vi "XML - Get extra pages XML string.vi"(8 "error in (no error)":errorcluster, 9 "CD Template":refnum<class "NIVS_CD Template.lvclass">, 10 "Project Name":string, 11 "CD Wizard - Internal Data":T1) -> (0 "error out":errorcluster, 3 "Extra Pages XML string":string)   [LabVIEW 2016, in "NIVS_Consolidated_CDW_MetaDataObj.lvclass"]
doc: "Creates the XML section for the extra pages. VeriStand needs for each extra page a section in the XML file to know the extra page and the corresponding configuration for the extra page."
uses:
  NIVS_Consolidated_CDW_MetaDataObj.lvclass
  Internal data.ctl
  Template Classes/NIVS_CD Template/NIVS_CD Template.lvclass
  Template Classes/NIVS_CD Template/NIVS_CD Template.lvclass/NIVS_CD Template.ctl
  Template Classes/NIVS_CD Template/Read Extra Page Names.vi
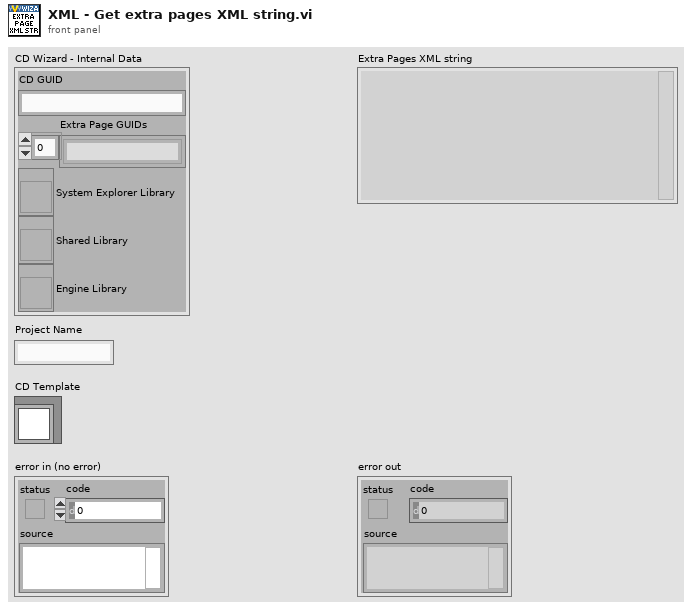
[diagram p1: front panel]
types:
  T1 = typedef "NIVS_Consolidated_CDW_MetaDataObj.lvclass/Internal data.ctl" = cluster{"CD GUID":string, "Extra Page GUIDs":string[], "System Explorer Library":refnum<vi>, "Shared Library":refnum<vi>, "Engine Library":refnum<vi>}
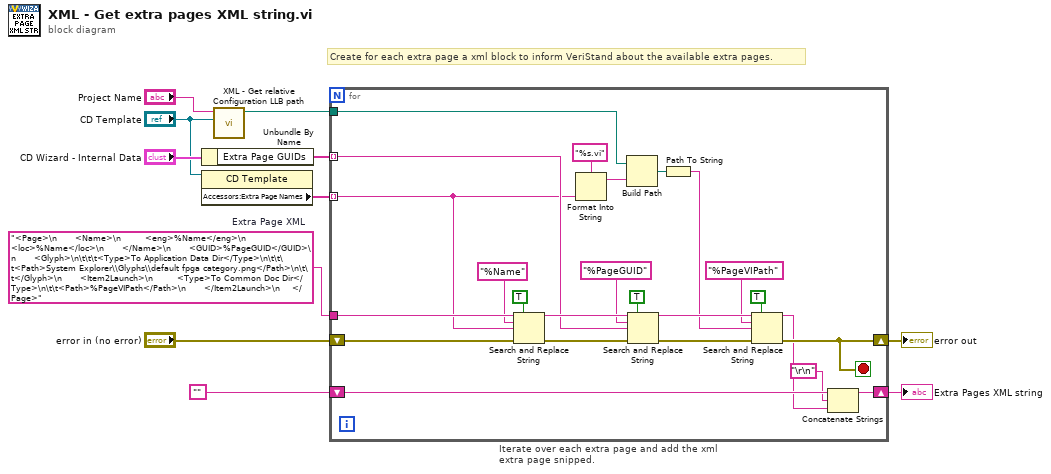
[diagram p0: block diagram]
diagram:
  w10 = "<Page>\n      <Name>\n        <eng>%Name</eng>\n        <loc>%Name</loc>\n      </Name>\n      <GUID>%PageGUID</GUID>\n      <Glyph>\n\t\t\t<Type>To Application Data Dir</Type>\n\t\t\t<Path>System Explorer\\Glyphs\\default fpga category.png</Path>\n\t\t</Glyph>\n      <Item2Launch>\n        <Type>To Common Doc Dir</Type>\n\t\t<Path>%PageVIPath</Path>\n      </Item2Launch>\n    </Page>"  # Extra Page XML
  # "Create for each extra page a xml block to inform VeriStand about the available extra pages."
  n1 = Unbundle By Name("CD Wizard - Internal Data") -> ("Extra Page GUIDs"=w4:string[])
  n2 = property class="CD Template"(reference="CD Template") -> ("Accessors:Extra Page Names"=w1:string[])  [unwired: 1 in, 2 out]
  n3 = call "XML - Get relative Configuration LLB path.vi"("CD Template"="CD Template", "Project Name"="Project Name") -> ("Relative Configuration LLB path"=w7:path)  [unwired: 9 in]
  n4 = for "Iterate over each extra page and add the xml extra page snipped." {
    tunnel: w10 -> [w35]
    shift-right: [w26] -> w9
    shift-left: "" -> [w25]
    shift-right: [w22] -> w11
    shift-left: "error in (no error)" -> [w23]
    tunnel: w7 -> [w18]
    tunnel: w4 -> [w14] mode=indexing
    tunnel: w1 -> [w13] mode=indexing
    stop <- w22 stop-if-true
    n5 = Search and Replace String(replace all?=TRUE ("replace all? (F)"), input string=w35, search string="%Name", replace string=w13, error in=w23) -> (result string=w31:string, error out=w24:errorcluster)  [unwired: 5 out]
    n6 = Format Into String(format string="%s.vi", w13) -> (resulting string=w17:string)  [unwired: 2 in, 1 out]
    n7 = Build Path(base path=w18, name or relative path=w17) -> (appended path=w20:path)
    n8 = Search and Replace String(replace all?=TRUE ("replace all? (F)"), input string=w31, search string="%PageGUID", replace string=w14, error in=w24) -> (result string=w28:string, error out=w12:errorcluster)  [unwired: 5 out]
    n9 = Path To String(path=w20) -> (string=w19:string)
    n10 = Search and Replace String(replace all?=TRUE ("replace all? (F)"), input string=w28, search string="%PageVIPath", replace string=w19, error in=w12) -> (result string=w15:string, error out=w22:errorcluster)  [unwired: 5 out]
    n11 = Concatenate Strings(w25, "\r\n", w15) -> (w26:string)
  }
  "error out" <- w11
  "Extra Pages XML string" <- w9
